vi "CreateVI.vi"(8 "error in (no error)":errorcluster, 11 "Wait Time (ms)":u32) -> (0 "error out":errorcluster, 3 "millisecond timer value":u32)   [LabVIEW 2017]
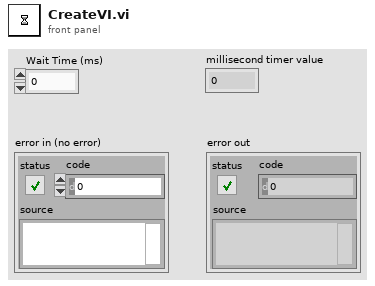
[diagram p1: front panel]
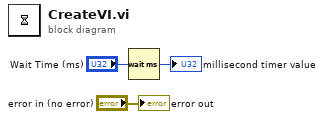
[diagram p0: block diagram]
diagram:
  n1 = Wait (ms)(milliseconds to wait="Wait Time (ms)") -> (millisecond timer value=→"millisecond timer value":u32)
  "error out" <- "error in (no error)"
